vi "StartVXM.vi"(11 "Stepper Controller Port":i32) -> (3 "String":string)   [LabVIEW 2020]
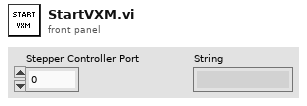
[diagram p1: front panel]
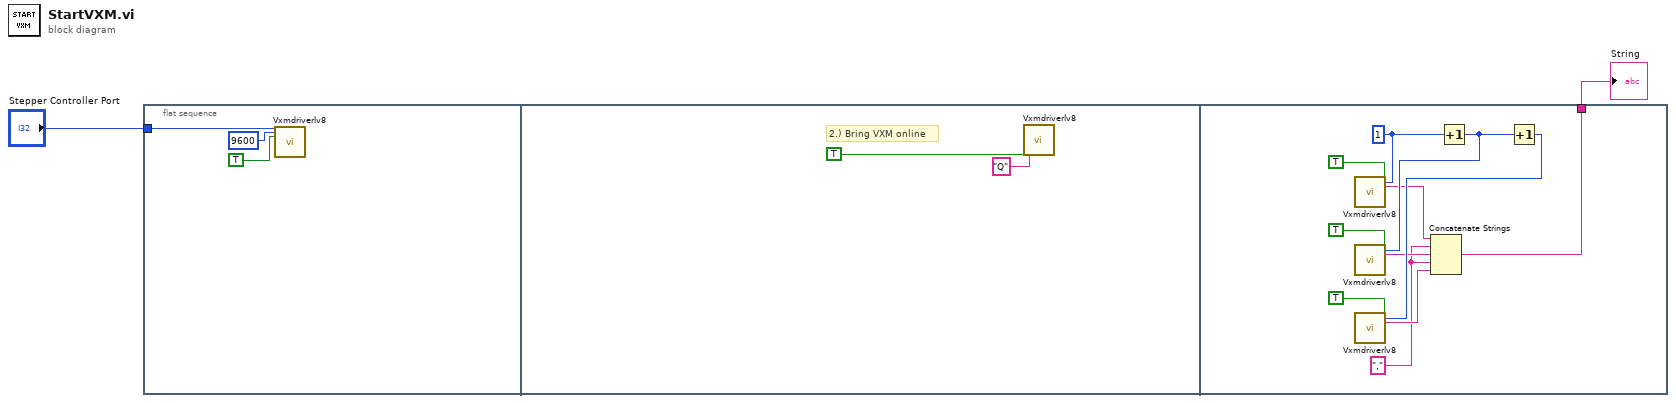
[diagram p0: block diagram]
diagram:
  n1 = flat-sequence {
    tunnel: "Stepper Controller Port" -> [w5]
    tunnel: [w8] -> w2
    frame #0 {
      n2 = call "Vxmdriverlv8.Vi"("Port"=w5, "Baud Rate"=9600, "Open Port"=TRUE) -> ()  [unwired: 19 in, 6 out]
    }
    frame #1 {
      # "2.) Bring VXM online"
      n3 = call "Vxmdriverlv8.Vi"("Send\nchars\nto port"=TRUE, "Chars to send"="Q") -> ()  [unwired: 20 in, 6 out]
    }
    frame #2 {
      w9 = ","
      w15 = 1 ("Motor\nNumber")
      n4 = call "Vxmdriverlv8.Vi"("Get\nMotor\nPosition"=TRUE ("Get\nMotor\nPosition"), "Motor\nNumber"=w15) -> ("Motor Position"=w12:string)  [unwired: 20 in, 5 out]
      n5 = Increment(x=w15) -> (x+1=w14:i32)
      n6 = call "Vxmdriverlv8.Vi"("Get\nMotor\nPosition"=TRUE ("Get\nMotor\nPosition"), "Motor\nNumber"=w14) -> ("Motor Position"=w11:string)  [unwired: 20 in, 5 out]
      n7 = Increment(x=w14) -> (x+1=w13:i32)
      n8 = call "Vxmdriverlv8.Vi"("Get\nMotor\nPosition"=TRUE ("Get\nMotor\nPosition"), "Motor\nNumber"=w13) -> ("Motor Position"=w10:string)  [unwired: 20 in, 5 out]
      n9 = Concatenate Strings(w12, w9, w11, w9, w10) -> (w8:string)
    }
  }
  "String" <- w2
